vi "Set Front Panel Origin.vi"(8 "错误输入":errorcluster, 10 "原点":T1 caption="点", 11 "VI Ref In":refnum<vi>) -> (0 "错误输出":errorcluster, 3 "VI Ref Out":refnum<vi>)   [LabVIEW 2012, in "VIRef.lvlib"]
uses:
  VIRef.lvlib
  <vilib>/Utility/miscctls.llb/LVPointTypeDef.ctl
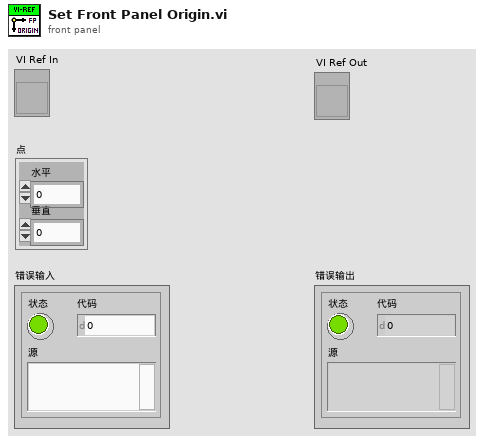
[diagram p1: front panel]
types:
  T1 = typedef "LVPointTypeDef.ctl" = cluster{"Horizontal":i16, "Vertical":i16}
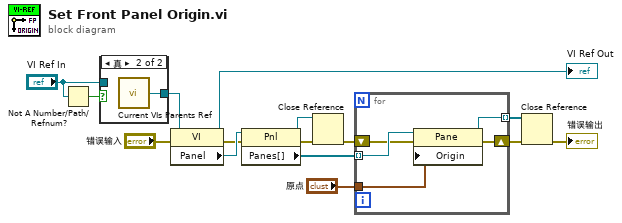
[diagram p0: block diagram]
diagram:
  n1 = Not A Number/Path/Refnum?(number/path/refnum="VI Ref In") -> (NaN/Path/Refnum?=w14:bool)
  n2 = case shown="真" w14 {
    tunnel: [w16 w17] -> w13
    tunnel: "VI Ref In" -> [w16 _]
    frame False {
    }
    frame True {
      n3 = call "Current VIs Parents Ref.vi"() -> ("Calling VI's Reference"=w17:refnum<vi>)  [unwired: 2 in]
    }
  }
  n4 = property class="VI"(reference=w13, error in="错误输入") -> (reference out=→"VI Ref Out":refnum<vi>, error out=w10:errorcluster, "Panel"=w11:refnum<vi>)
  n5 = property class="Pnl"(reference=w11, error in=w10) -> (reference out=w7:refnum<vi>, error out=w8:errorcluster, "Panes[]"=w6:refnum<vi>[])
  n6 = Close Reference(reference=w7, error in (no error)=w8) -> (error out=w5:errorcluster)
  n7 = for {
    tunnel: w6 -> [w22] mode=indexing
    shift-right: [w20] -> w4
    shift-left: w5 -> [w21]
    tunnel: [w19] -> w3 mode=indexing
    tunnel: "原点" -> [w18]
    n8 = property class="Pane"(reference=w22, error in=w21, "Origin"=w18) -> (reference out=w19:refnum<vi>, error out=w20:errorcluster)
  }
  n9 = Close Reference(reference=w3, error in (no error)=w4) -> (error out=→"错误输出":errorcluster)
